vi "Background Gradient SLM.vi"(2 "Action":u16(ring) items=["Read", "Initialize"]) -> (6 "gradient":dbl[][](array[numeric]), 10 "holo mask":dbl[][](array[numeric]))   [LabVIEW 2014]
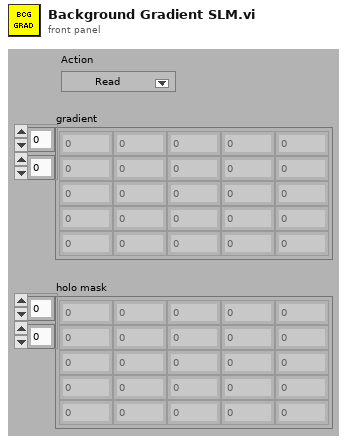
[diagram p1: front panel]
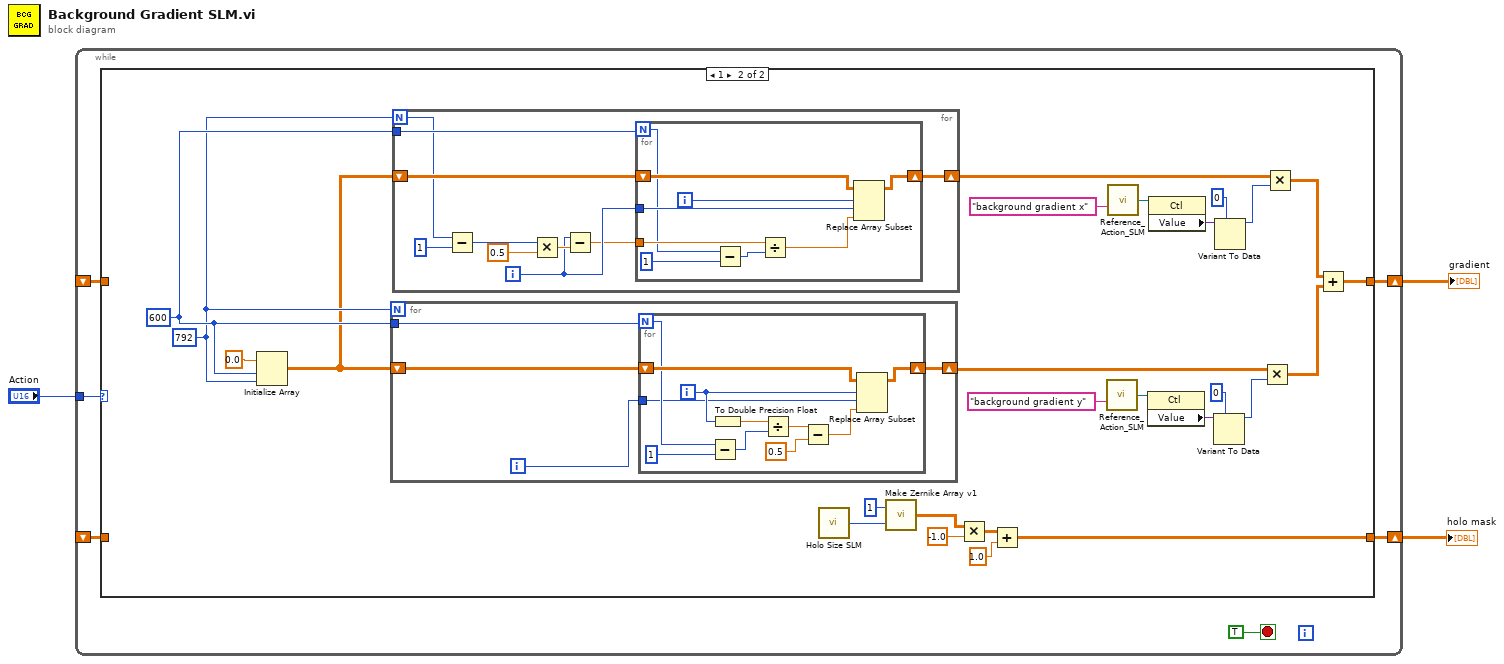
[diagram p0: block diagram]
diagram:
  n1 = while {
    shift-right: [w6] -> w2
    shift-left: _ -> [w7]
    tunnel: "Action" -> [w8]
    shift-right: [w5] -> w1
    shift-left: _ -> [w4]
    stop <- TRUE stop-if-true
    n2 = case shown="1" w8 {
      tunnel: w7 -> [w11 _]
      tunnel: [w11 w28] -> w6
      tunnel: [w10 w12] -> w5
      tunnel: w4 -> [w10 _]
      frame 0, Default {
      }
      frame 1 {
        w36 = 792 ("dimension size")
        w37 = 600
        n3 = Initialize Array(0.0 ("element"), w37, w36) -> (w35:dbl[][])
        n4 = for {
          N: w36 -> [_]
          tunnel: w37 -> [w59]
          shift-right: [w58] -> w15
          shift-left: w35 -> [w60]
          i -> [w57]
          n5 = for {
            N: w59 -> [w63]
            shift-right: [w70] -> w58
            shift-left: w60 -> [w69]
            tunnel: w57 -> [w61]
            i -> [w71]
            n6 = Subtract(x=w63, y=1) -> (x-y=w64:i32)
            n7 = To Double Precision Float(number=w71) -> (double precision float=w68:dbl)
            n8 = Divide(x=w68, y=w64) -> (x/y=w66:dbl)
            n9 = Subtract(x=w66, y=0.5 ("element")) -> (x-y=w65:dbl)
            n10 = Replace Array Subset(array=w69, new element=w65, index (row)=w71, index (col)=w61) -> (w70:dbl[][])
          }
        }
        n11 = for {
          N: w36 -> [w40]
          tunnel: w37 -> [w46]
          shift-right: [w45] -> w21
          shift-left: w35 -> [w47]
          i -> [w42]
          n12 = Subtract(x=w40, y=1) -> (x-y=w39:i32)
          n13 = Multiply(x=w39, y=0.5 ("element")) -> (x*y=w43:dbl)
          n14 = Subtract(x=w42, y=w43) -> (x-y=w41:dbl)
          n15 = for {
            N: w46 -> [w49]
            shift-right: [w55] -> w45
            shift-left: w47 -> [w54]
            tunnel: w42 -> [w53]
            tunnel: w41 -> [w52]
            i -> [w56]
            n16 = Subtract(x=w49, y=1) -> (x-y=w48:i32)
            n17 = Divide(x=w52, y=w48) -> (x/y=w51:dbl)
            n18 = Replace Array Subset(array=w54, new element=w51, index (row)=w56, index (col)=w53) -> (w55:dbl[][])
          }
        }
        n19 = call "Holo Size SLM.vi"() -> ("data"=w27:i32)  [unwired: 15 in]
        n20 = call "Make Zernike Array v1.vi"("size"=w27, "z"=u8 1) -> ("zernike array"=w31:dbl[][])
        n21 = Multiply(x=w31, y=-1.0) -> (x*y=w30:dbl[][])
        n22 = Add(x=w30, y=1.0) -> (x+y=w28:dbl[][])
        n23 = call "Reference_Action_SLM.vi"("Control Name"="background gradient y") -> ("Ref OUT"=w19:refnum<vi>)  [unwired: 12 in, 2 out]
        n24 = call "Reference_Action_SLM.vi"("Control Name"="background gradient x") -> ("Ref OUT"=w25:refnum<vi>)  [unwired: 12 in, 2 out]
        n25 = property class="Ctl"(reference=w19) -> ("Value"=w18:variant)  [unwired: 1 in, 2 out]
        n26 = property class="Ctl"(reference=w25) -> ("Value"=w24:variant)  [unwired: 1 in, 2 out]
        n27 = Variant To Data(type=0, Variant=w18) -> (data=w16:i32)  [unwired: 1 in, 1 out]
        n28 = Variant To Data(type=0, Variant=w24) -> (data=w22:i32)  [unwired: 1 in, 1 out]
        n29 = Multiply(x=w15, y=w16) -> (x*y=w13:dbl[][])
        n30 = Multiply(x=w21, y=w22) -> (x*y=w14:dbl[][])
        n31 = Add(x=w14, y=w13) -> (x+y=w12:dbl[][])
      }
    }
  }
  "holo mask" <- w2
  "gradient" <- w1
